vi "GLOBALDriver.vi"() -> ()   [LabVIEW 2011]
uses:
  <vilib>/Rock Robotics/WPI/Joystick/WPI_JoystickButtonState.ctl
panel:
  out "Joystick 3 B":T1
  out "Joystick 3 A":T2
  out "Shooter Slider":dbl
  out "Right Foot Pedal":bool
  out "Left Foot Pedal":bool
  out "Joystick 2 B":T1
  out "Joystick 2 A":T2
  out "Joystick 1 B":T1
  out "Joystick 1 A":T2
  in  "Right HighRes Button":bool
  out "Left HighRes Button":bool
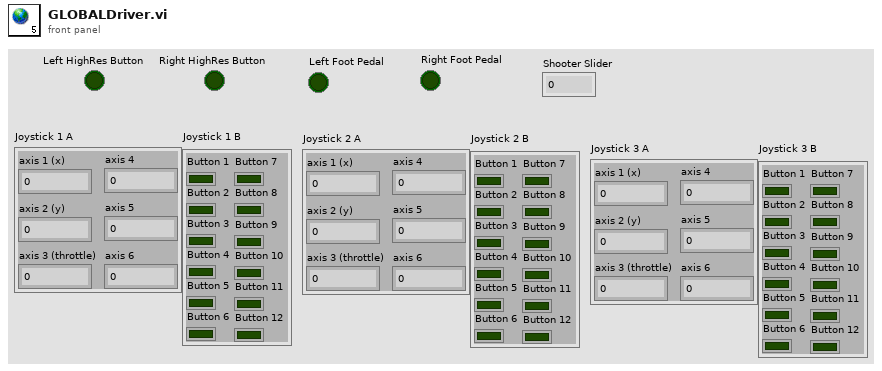
[diagram p1: front panel]
types:
  T1 = typedef "WPI_JoystickButtonState.ctl" = cluster{"Button 1":bool, "Button 2":bool, "Button 3":bool, "Button 4":bool, "Button 5":bool, "Button 6":bool, "Button 7":bool, "Button 8":bool, "Button 9":bool, "Button 10":bool, "Button 11":bool, "Button 12":bool}
  T2 = cluster{"axis 1 (x)":dbl, "axis 2 (y)":dbl, "axis 3 (throttle)":dbl, "axis 4":dbl, "axis 5":dbl, "axis 6":dbl}
diagram:
